vi "rql_Listen for Data.vi"(8 "error in":errorcluster, 9 "Data in":T1, 11 "DS TCP Read in":refnum<class "DS TCP Read.lvclass">) -> (0 "error out":errorcluster, 3 "dup DS TCP Read out":refnum<class "DS TCP Read.lvclass">)   [LabVIEW 2017, in "DS TCP Server.lvlib" / "DS TCP Read.lvclass"]
doc: "This VI sends a <b>Local API Request</b> message to an MHL case of the Worker that owns this VI.\n---\nContinously wait and read data from a Debug Client. Forward this data directly to either the Application Manager Worker or a Message Log Worker."
uses:
  DS TCP Read.lvclass
  C:/Program Files (x86)/National Instruments/LabVIEW 2017/vi.lib/addons/_Workers/Library/Classes/Worker/Worker.lvclass
  rql_Listen for Data.ctl
  <vilib>/addons/_Workers/Library/Classes/Message/Priority.ctl
  <vilib>/addons/_Workers/Library/Classes/Message/Enqueue Message to Self v2.vi
  <vilib>/addons/_Workers/Library/Classes/Message/Message.lvclass
  C:/Program Files (x86)/National Instruments/LabVIEW 2017/vi.lib/addons/_Workers/Library/Classes/Workers Object/Workers Object.lvclass
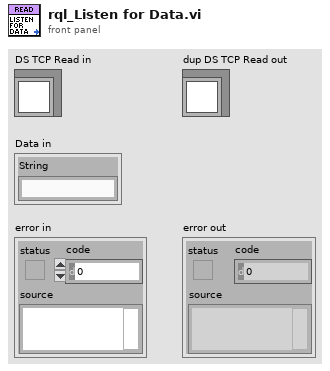
[diagram p1: front panel]
types:
  T1 = typedef "DS TCP Server.lvlib/DS TCP Read.lvclass/rql_Listen for Data.ctl" = cluster{"String":string}
  T2 = typedef "Workers.lvlib/Message.lvclass/Priority.ctl" = enum16{"Low", "Normal", "High"}
  T3 = typedef "Workers.lvlib/Case Label.ctl" = string
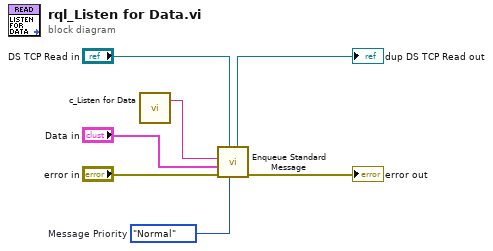
[diagram p0: block diagram]
diagram:
  w5 = Priority."Normal"  # Message Priority
  n1 = call "c_Listen for Data.vi"() -> ("Case Label"=w4:T3)  [unwired: 1 in]
  n2 = call-poly <vilib>:"Enqueue Standard Message.vi"("Priority (Normal)"=w5, "Worker"="DS TCP Read in", "error in"="error in", "Data"="Data in", "Case Label"=w4) -> ("error out"=→"error out":errorcluster, "dup Worker out"=→"dup DS TCP Read out":refnum<class "DS TCP Read.lvclass">)  [unwired: 5 in]
